vi "LlenarVoltajeTabla.vi"(7 "fila":i32, 10 "Dato":string, 11 "Tabla in":string[][](array[string])) -> (3 "Tabla out":string[][](array[string]))   [LabVIEW 2019, in "Prueba05.lvclass"]
uses:
  Prueba05.lvclass
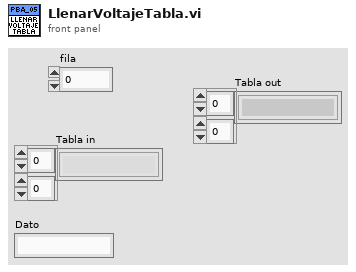
[diagram p1: front panel]
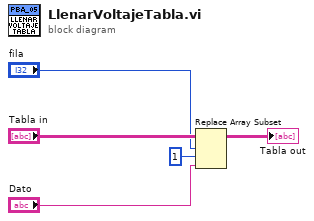
[diagram p0: block diagram]
diagram:
  n1 = Replace Array Subset(array="Tabla in", new element="Dato", index (row)="fila", index (col)=1 ("disabled index (col)")) -> (→"Tabla out":string[][])
